vi "Write EST Tunnel.vi"(8 "error in (no error)":errorcluster, 10 "EST Tunnel":refnum<vi>, 11 "IO Loop in":refnum<class "Module Loop.lvclass">) -> (0 "error out":errorcluster, 3 "IO Loop out":refnum<class "Module Loop.lvclass">)   [LabVIEW 2015, in "Module Loop.lvclass"]
uses:
  Module Loop.lvclass
  Module Loop.lvclass/Module Loop.ctl
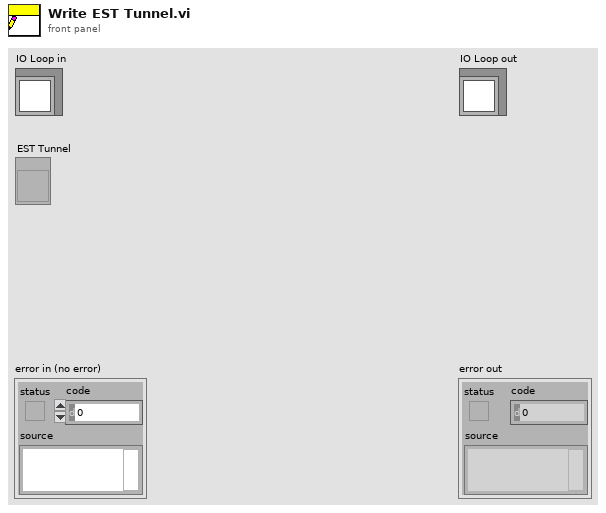
[diagram p1: front panel]
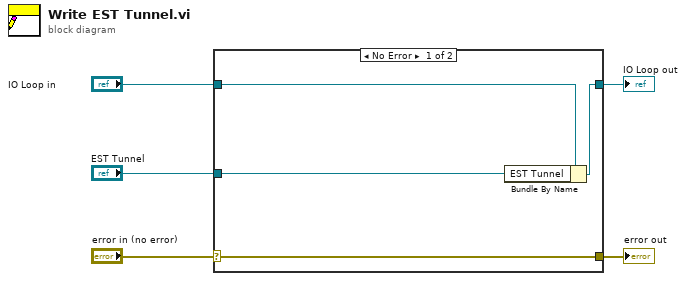
[diagram p0: block diagram]
diagram:
  n1 = case shown="No Error" "error in (no error)" {
    selector: "error in (no error)" -> [w9 w10]
    tunnel: [w9 w10] -> w4
    tunnel: [w7 w11] -> w2
    tunnel: "IO Loop in" -> [w8 w11]
    tunnel: "EST Tunnel" -> [w6 _]
    frame No Error {
      n2 = Bundle By Name(cluster=w8, "EST Tunnel"=w6) -> (w7:refnum<class "Module Loop.lvclass">)
    }
    frame Error {
    }
  }
  "error out" <- w4
  "IO Loop out" <- w2
